vi "SimpleListSelection.vi"(6 "Timeout (-1)":i32=-1, 7 "Blacken (F)":bool, 8 "error in":errorcluster, 9 "Selection Mode":T1, 10 "Items List":string[](array[string]), 11 "Message":string) -> (0 "error out":errorcluster, 1 "Selection":i32[](array[numeric]), 2 "Items List dup":string[](array[string]), 3 "First Element":i32, 4 "cancelled":bool)   [LabVIEW 2012]
uses:
  ListSelection/Selection Mode.ctl
  ListSelection/ListSelection.lvclass
  ListSelection/ListSelection.lvclass/ListSelection.ctl
  Dialog/Dialog/Dialog.lvclass/Dialog.ctl
  Dialog/Dialog/Dialog.lvclass
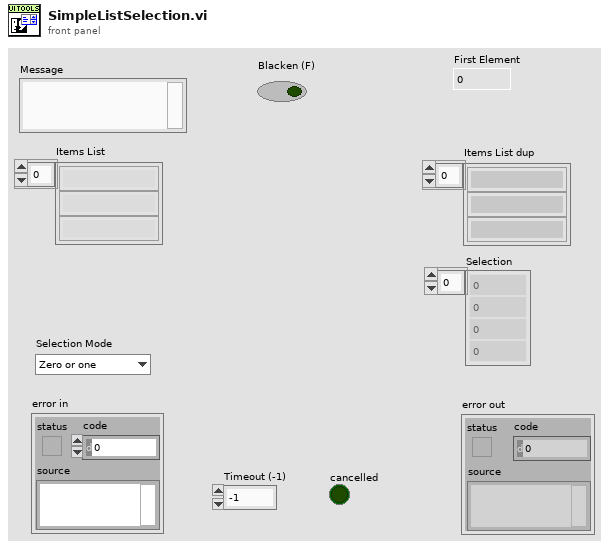
[diagram p1: front panel]
types:
  T1 = typedef "ListSelection.lvlib/ListSelection.lvclass/Selection Mode.ctl" = enum16{"Zero or one", "One", "Zero or more", "One or more"}
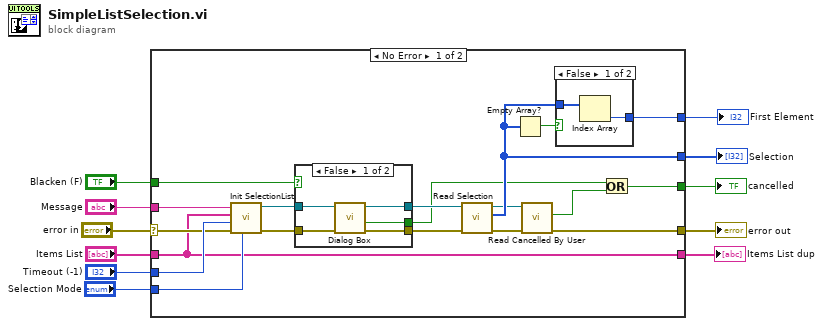
[diagram p0: block diagram]
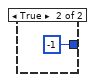
[diagram p2: hidden frame]
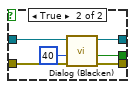
[diagram p3: hidden frame]
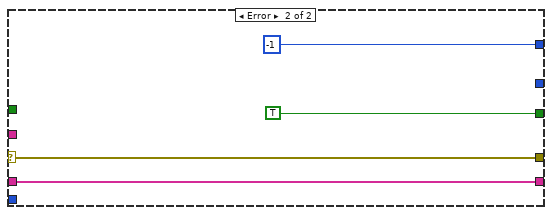
[diagram p4: hidden frame]
diagram:
  n1 = case shown="No Error" "error in" {
    selector: "error in" -> [w22 w47]
    tunnel: [w12 TRUE] -> w11
    tunnel: [w15 w47] -> w10
    tunnel: "Blacken (F)" -> [w30 _]
    tunnel: "Message" -> [w29 _]
    tunnel: "Items List" -> [w21 w46]
    tunnel: "Timeout (-1)" -> [w28 _]
    tunnel: "Selection Mode" -> [w25 _]
    tunnel: [w24 -1] -> w5
    tunnel: [w19 _] -> w4
    tunnel: [w21 w46] -> w1
    frame No Error {
      n2 = call "Init SelectionList.vi"("Selection Mode"=w25, "error in"=w22, "Timeout (-1)"=w28, "Items List"=w21, "Message"=w29) -> ("error out"=w26:errorcluster, "ListSelection out"=w27:refnum<class "ListSelection.lvclass">)  [unwired: 5 in]
      n3 = case shown="False" w30 {
        tunnel: w27 -> [w38 w44]
        tunnel: w26 -> [w37 w43]
        tunnel: [w36 w40] -> w14
        tunnel: [w35 w41] -> w18
        tunnel: [w34 w39] -> w20
        frame False {
          n4 = call-dynamic "Dialog Box.vi"("error in (no error)"=w37, "Msg_Error in"=w38) -> ("error out"=w35:errorcluster, "timed out?"=w36:bool, "Msg_Error out"=w34:refnum<class "ListSelection.lvclass">)  [unwired: 6 in, 1 out]
        }
        frame True {
          n5 = call-dynamic "Dialog (Blacken).vi"("error in (no error)"=w43, "Transparency (40)"=u8 40, "Dialog in"=w44) -> ("error out"=w41:errorcluster, "timed out?"=w40:bool, "Dialog out"=w39:refnum<class "ListSelection.lvclass">)  [unwired: 5 in, 1 out]
        }
      }
      n6 = call "Read Selection.vi"("error in (no error)"=w18, "ListSelection in"=w20) -> ("error out"=w16:errorcluster, "Selection"=w19:i32[], "ListSelection out"=w17:refnum<class "ListSelection.lvclass">)  [unwired: 7 in]
      n7 = Empty Array?(array=w19) -> (empty?=w23:bool)
      n8 = call "Read Cancelled By User.vi"("error in (no error)"=w16, "Dialog in"=w17) -> ("error out"=w15:errorcluster, "cancelled by user?"=w13:bool)  [unwired: 7 in, 1 out]
      n9 = case shown="False" w23 {
        tunnel: [w32 -1] -> w24
        tunnel: w19 -> [w31 _]
        frame False {
          n10 = Index Array(array=w31) -> (element=w32:i32)  [unwired: 1 in]
        }
        frame True {
        }
      }
      n11 = Or(x=w14, y=w13) -> (x .or. y?=w12:bool)
    }
    frame Error {
    }
  }
  "cancelled" <- w11
  "error out" <- w10
  "Items List dup" <- w1
  "Selection" <- w4
  "First Element" <- w5
